vi "Main_UI.vi"(8 "error in (no error)":errorcluster) -> (0 "error out":errorcluster)   [LabVIEW 2019]
uses:
  Ctrl/SwitchBtn.ctl
  <vilib>/Utility/miscctls.llb/LVPointTypeDef.ctl
  <vilib>/Utility/miscctls.llb/LVPositionTypeDef.ctl
  Function/Main UI/Glb/Main_UI Gb.vi
  LLB/Commonly VI.lvlib
panel:
  in  "Tab Control":enum32{"Page 1", "Page 2"}(tab)
  in  "StopReceiveCmd":T1 caption="停止接收外部命令"
  in  "Tab Control 2":enum32{"動作流程", "檢測結果"}(tab)
  in  "ProcessList":i32(listbox) caption="動作流程"
  out "Result Arr":T2(array[cluster]) caption="結果列表"
  out "VirbConnect":bool caption="震動盤連接"
  out "Connected":bool caption="通訊連線"
  out "Image":T3(plugin-control)
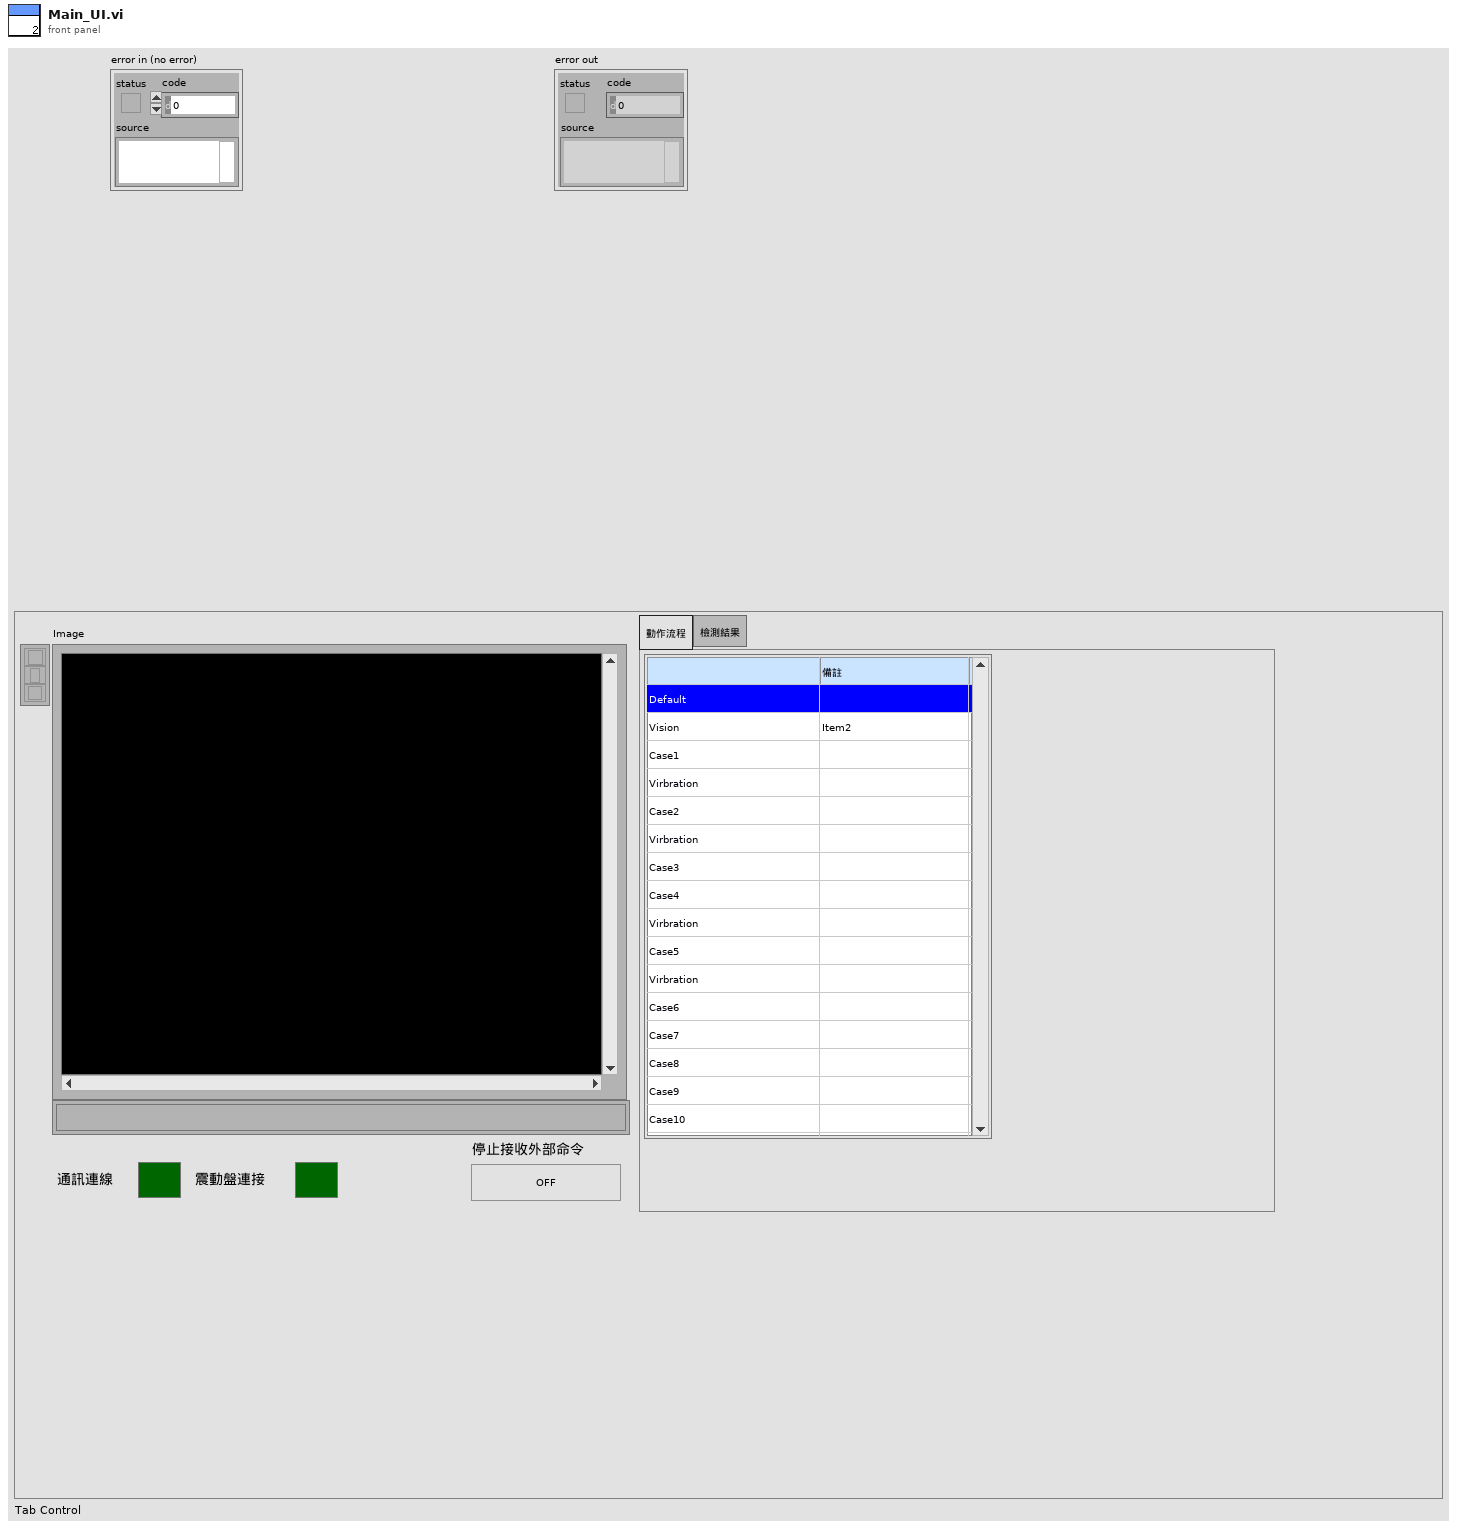
[diagram p1: front panel]
types:
  T1 = typedef "SwitchBtn.ctl" = bool
  T2 = cluster{"ROI":string, "Numbers":i32, "Data":string[][]}[]
  T3 = typedef "IMAQ Image.ctl" = refnum<image>
  T4 = typedef "LVPositionTypeDef.ctl" = cluster{"Left":i32, "Top":i32}
  T5 = typedef "LVPointTypeDef.ctl" = cluster{"Horizontal":i16, "Vertical":i16}
  T6 = enum16{"Initial", "Write", "Read", "Save", "Load", "WrteAll"}
  T7 = cluster{"ProcessList":refnum<vi>, "Result Arr":refnum<vi>, "StopReceiveCmd":refnum<vi>}
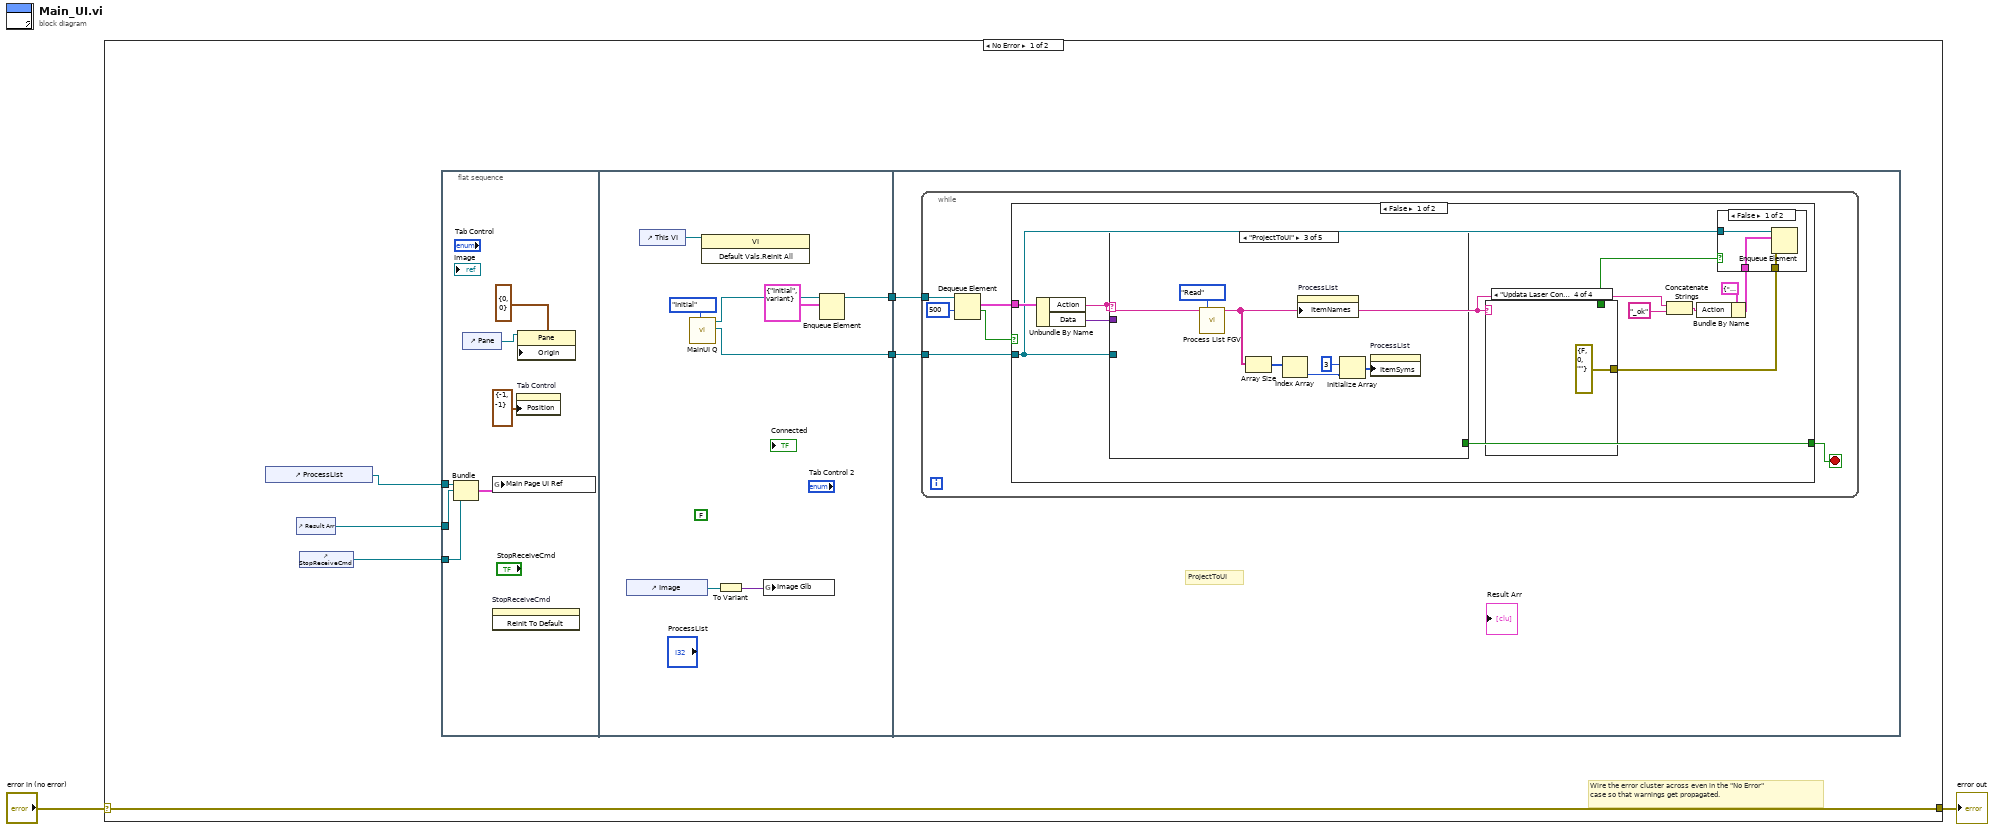
[diagram p0: block diagram]
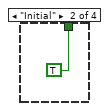
[diagram p4: hidden frame]
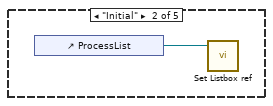
[diagram p7: hidden frame]
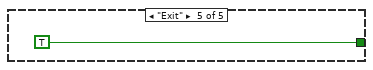
[diagram p9: hidden frame]
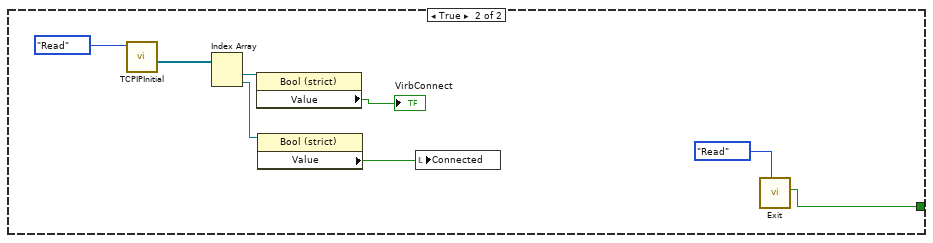
[diagram p10: hidden frame]
diagram:
  n1 = case shown="No Error" "error in (no error)" {
    selector: "error in (no error)" -> [w8 w64]
    tunnel: [w8 w64] -> w1
    frame No Error {
      # "Wire the error cluster across even in the \"No Error\"\ncase so that warnings get propagated."
      n2 = control-ref of="ProcessList"() -> (w5:refnum<vi>)
      n3 = control-ref of="Result Arr"() -> (w4:refnum<vi>)
      n4 = control-ref of="StopReceiveCmd"() -> (w3:refnum<vi>)
      n5 = flat-sequence {
        tunnel: w5 -> [w15]
        tunnel: w4 -> [w10]
        tunnel: w3 -> [w9]
        tunnel: [w23] -> w7
        tunnel: [w18] -> w6
        tunnel: w7 -> [w25]
        tunnel: w6 -> [w24]
        frame #0 {
          n6 = Bundle("ProcessList"=w15, "Result Arr"=w10, "StopReceiveCmd"=w9) -> (w11:T7)  [unwired: 1 in]
          n7 = control-ref of="Pane"() -> (w14:refnum<vi>)
          n8 = global write "Main_UI Gb.vi" "Main Page UI Ref"(w11) -> ()
          n9 = invoke on="StopReceiveCmd" class="Bool (strict)" method="Reinit To Default"() -> ()  [unwired: 3 in, 3 out]
          n10 = property on="Tab Control" class="TabCtl (strict)"("Position"=T4 {"Left"=-1, "Top"=-1}) -> ()  [unwired: 2 in, 2 out]
          n11 = property class="Pane"(reference=w14, "Origin"=T5 {"Horizontal"=0, "Vertical"=0}) -> ()  [unwired: 1 in, 2 out]
        }
        frame #1 {
          (unwired) FALSE ("Reply pause")
          n12 = control-ref of="Image"() -> (w17:refnum<vi>)
          n13 = control-ref of="This VI"() -> (w21:refnum<vi>)
          n14 = call "MainUI Q.vi"("Enum"=enum16{"Initial", "read", "release"}."Initial") -> ("UI Response Out"=w18:refnum<queue>, "UI Receive Out"=w19:refnum<queue>)  [unwired: 9 in]
          n15 = invoke class="VI" method="Default Vals.Reinit All"(reference=w21) -> ()  [unwired: 2 in, 3 out]
          n16 = To Variant(anything=w17) -> (Variant=w16:variant)
          n17 = global write "Main_UI Gb.vi" "Image Glb"(w16) -> ()
          n18 = Enqueue Element(queue=w19, element=cluster{"Action":string, "Data":variant} {"Action"="Initial", "Data"=variant}) -> (queue out=w23:refnum<queue>)  [unwired: 2 in, 2 out]
        }
        frame #2 {
          # "ProjectToUI"
          n19 = while {
            tunnel: w25 -> [w31]
            tunnel: w24 -> [w29]
            stop <- w28 stop-if-true
            n20 = Dequeue Element(queue=w31, timeout in ms (-1)=500) -> (element=w30:cluster{"Action":string, "Data":variant}, timed out?=w27:bool)  [unwired: 1 in, 2 out]
            n21 = case shown="False" w27 {
              tunnel: w30 -> [w42 _]
              tunnel: w29 -> [w39 _]
              tunnel: [w41 w63] -> w28
              frame False {
                n22 = Unbundle By Name(w42) -> ("Action"=w35:string, "Data"=w40:variant)
                n23 = case shown="\"ProjectToUI\"" w35 {
                  tunnel: w39 -> [_ _ _ _ _]
                  tunnel: [_ _ _ _ TRUE] -> w41
                  tunnel: w40 -> [_ _ _ _ _]
                  frame "False", Default {
                  }
                  frame "Initial" {
                    n24 = control-ref of="ProcessList"() -> (w48:refnum<vi>)
                    n25 = call "Set Listbox ref.vi"("ListRef"=w48) -> ()  [unwired: 10 in, 1 out]
                  }
                  frame "ProjectToUI" {
                    n26 = call "Process List FGV.vi"("Action"=T6."Read") -> ("TableOut"=w53:string[][])  [unwired: 12 in, 2 out]
                    n27 = Array Size(array=w53) -> (size(s)=w52:i32[])
                    n28 = Index Array(array=w52) -> (element=w51:i32)  [unwired: 1 in]
                    n29 = property on="ProcessList" class="MCListbox (strict)"("ItemNames"=w53) -> ()  [unwired: 2 in, 2 out]
                    n30 = Initialize Array(3 ("element"), w51) -> (w50:i32[])
                    n31 = property on="ProcessList" class="MCListbox (strict)"("ItemSyms"=w50) -> ()  [unwired: 2 in, 2 out]
                  }
                  frame "SetSyms" {
                  }
                  frame "Exit" {
                  }
                }
                n32 = case shown="\"Updata Laser Connect\"" w35 {
                  tunnel: [_ _ _ errorcluster {"status"=FALSE, "code"=0, "source"=""} ("error constant")] -> w33
                  tunnel: [_ TRUE _ _] -> w32
                  frame "False", Default {
                  }
                  frame "Initial" {
                  }
                  frame "ProjectToUI" {
                  }
                  frame "Updata Laser Connect" {
                  }
                }
                n33 = Concatenate Strings(w35, "_ok" ("string")) -> (w36:string)
                n34 = Bundle By Name(cluster=cluster{"Action":string, "Data":variant} {"Action"="", "Data"=variant} ("element"), "Action"=w36) -> (w37:cluster{"Action":string, "Data":variant})
                n35 = case shown="False" w32 {
                  tunnel: w39 -> [w45 _]
                  tunnel: w37 -> [w44 _]
                  tunnel: w33 -> [w43 _]
                  frame False {
                    n36 = Enqueue Element(queue=w45, element=w44, error in (no error)=w43) -> ()  [unwired: 1 in, 3 out]
                  }
                  frame True {
                  }
                }
              }
              frame True {
                n37 = call "TCPIPInitial.vi"("Enum"=enum16{"initial", "Read", "release"}."Read") -> ("Connect"=w60:refnum<vi>[])  [unwired: 7 in, 3 out]
                n38 = Index Array(array=w60) -> (element #1=w59:refnum<vi>, element #2=w57:refnum<vi>)  [unwired: 2 in]
                n39 = property class="Bool (strict)"(reference=w59) -> ("Value"=→"VirbConnect":bool)  [unwired: 1 in, 2 out]
                n40 = property class="Bool (strict)"(reference=w57) -> ("Value"=w56:bool)  [unwired: 1 in, 2 out]
                n41 = local write "Connected"(w56) -> ()
                n42 = call "Exit.vi"("Enum"=enum16{"Initial", "Read", "Write"}."Read") -> ("ExitOut"=w63:bool)  [unwired: 10 in]
              }
            }
          }
        }
      }
    }
    frame Error {
    }
  }
  "error out" <- w1
